vi "PreviewCell.vi"(6 "Current Variable settings":T2[](array[typedef]), 9 "Col header":string, 10 "Line Timing":T1, 11 "Cell contents":string) -> ()   [LabVIEW 2013]
uses:
  TypeDefs/Active procedure variables.ctl
  TypeDefs/LineTiming.ctl
  PackedLibraries/LuaEvaluatorAPI.lvlibp/API/t_Caching_Expression_Evaluator_Methods_Table.ctl
  PackedLibraries/LuaEvaluatorAPI.lvlibp
panel:
  out "parsed dt":dbl format="%#_6p"
  out "actual dt=t/steps":dbl format="%#_6p"
  in  "error in (no error)":errorcluster
  out "error out":errorcluster
  in  "Stand-Alone?":bool caption="This should NOT be set when VI called externally.\nIt is only included for debugging. (Caller list is checked and functions below won't be defined if not empty)."
  in  "User defined functions (IF Stand-Alone)":string="----------------------------------------\n-- The following functions are part of the \"standard load\" of functions and should not be messed with\n-- They are here for reference only.\n-- Please add any user functions above this comment\n-- -------------------------------------------------------------------------------------------\n\n-- Creates a linear ramp from A to B\nfunction LineRamp(f, Initial, Final)\n    return (1-f)*Initial + f*Final;\nend\n\n-- Creates an exponential ramp from A to B\nfunction ExpRamp(t, a, b, tau)\n   return (b - a*exp(tMax / tau) + (a-b)*exp(t/tau))/ ( 1 - exp(tMax / tau) );\nend\n\n-- Creates a sinewave\nfunction SinRamp(t,Offset,A,Freq, Phase)\n    return Offset + A * sin(2*pi*Freq*t + Phase)\nend\n\n-- Creates a blackman pulse\nfunction Blackman(f, Offset, A)\n    return Offset +  A*sqrt(0.5*cos(3.1415*(2*f-1))+0.08*cos(2*pi*(2*f-1))+0.42);\nend\n\n-- Creates a half-gauss ramp\nfunction HalfGaussRamp(t, a, b, Width)\n    local y;\n    y = exp(-(tMax^2)/Width^2);\n    y = (a -  b*y)/(1-y)  +  ((b-a)/(1-y))*exp(-((t-tMax)^2)/Width^2);\n    return y;\nend\n\n-- Creates an \"O'Hara\" ramp from A to B, for dipole evaporation\nfunction EvapRamp(t, a, b, tau)\n   local y;\n  y = log(a/b) / log(1+tMax/tau);\n  y = a * (1+t/tau)^(-y);\n  return y;\nend\n\n----------------------------------------------------------------\n\n\n-- Creates an exponential ramp from A to B in tEnd seconds\n-- useful for stopping a ramp at different times to measure T, N\nfunction ExpRampStep(t, a, b, tau, tEnd)\n   return (b - a*exp(tEnd / tau) + (a-b)*exp(t/tau))/ ( 1 - exp(tEnd / tau) );\nend\n\nfunction ExpRampEnd(tEv, a, b, tau, tEnd)\n   return (b - a*exp(tEnd / tau) + (a-b)*exp(tEv/tau))/ ( 1 - exp(tEnd / tau) );\nend\n\nfunction ExpRamp2(t,a,tau)\n   return a*exp(-t/tau)\nend\n\nfunction ExpRamp2End(tEnd,a,tau)\n   return a*exp(-tEnd/tau)\nend"
  out "y values":dbl[](array[numeric])
  out "x values":dbl[](array[numeric])
  out "Group enabled?":bool
  out "Cell contents":string
  out "Waveform Graph":waveform(dbl)(graph)
  # "useful to indicate (row,col)?"
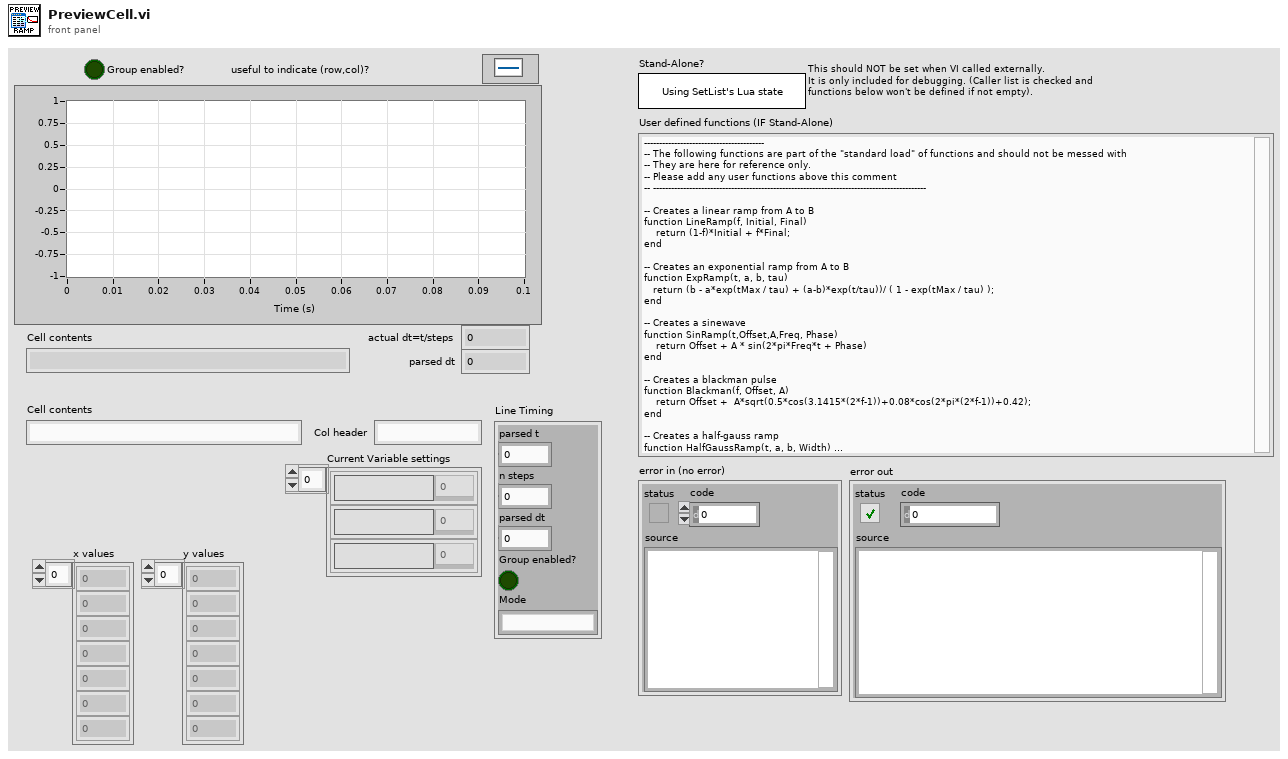
[diagram p1: front panel]
types:
  T1 = typedef "LineTiming.ctl" = cluster{"parsed t":dbl, "n steps":i32, "parsed dt":dbl, "Group enabled?":bool, "Mode":string}
  T2 = typedef "Active procedure variables.ctl" = cluster{"Procedure variable":string, "Value":dbl}
  T3 = typedef "LuaEvaluatorAPI.lvlibp/t_Caching_Expression_Evaluator_Methods_Table.ctl" = enum16{"set", "get", "eval", "assign", "isvalid", "execute", "evaltable", "close"}
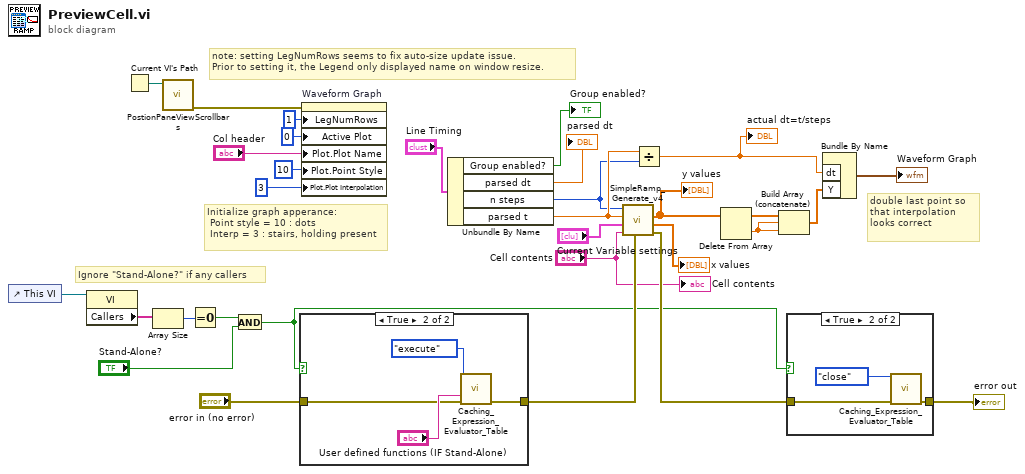
[diagram p0: block diagram]
diagram:
  # "note: setting LegNumRows seems to fix auto-size update issue.\nPrior to setting it, the Legend only displayed name on window resize."
  # "Ignore \"Stand-Alone?\" if any callers"
  # "Initialize graph apperance:\n Point style = 10 : dots\n Interp = 3 : stairs, holding present"
  # "double last point so that interpolation looks correct"
  n1 = control-ref of="This VI"() -> (w15:refnum<vi>)
  n2 = property class="VI"(reference=w15) -> ("Callers"=w14:string[])  [unwired: 1 in, 2 out]
  n3 = Current VI's Path() -> (path=w8:path)
  n4 = Array Size(array=w14) -> (size(s)=w13:i32)
  n5 = call "PostionPaneViewScrollbars.vi"("vi path"=w8) -> ("error out"=w7:errorcluster)  [unwired: 10 in]
  n6 = Equal To 0?(x=w13) -> (x = 0?=w12:bool)
  n7 = And(x=w12, y="Stand-Alone?") -> (x .and. y?=w10:bool)
  n8 = case shown="True" w10 {
    tunnel: [w32 w34] -> w29
    tunnel: "error in (no error)" -> [w32 w33]
    frame False {
    }
    frame True {
      n9 = call "Caching_Expression_Evaluator_Table.vi"("method"=t_Caching_Expression_Evaluator_Methods_Table."execute", "expression/scriptlet"="User defined functions (IF Stand-Alone)", "error in (no error)"=w33) -> ("error out"=w34:errorcluster)  [unwired: 10 in, 2 out]
    }
  }
  n10 = property on="Waveform Graph" class="WFGraph (strict)"(error in=w7, "LegNumRows"=u32 1 ("Active Plot"), "Active Plot"=u32 0, "Plot.Plot Name"="Col header", "Plot.Point Style"=u8 10, "Plot.Plot Interpolation"=u8 3) -> ()  [unwired: 1 in, 2 out]
  n11 = Unbundle By Name("Line Timing") -> ("Group enabled?"=→"Group enabled?":bool, "parsed dt"=→"parsed dt":dbl, "n steps"=w4:i32, "parsed t"=w5:dbl)
  n12 = call "SimpleRamp_Generate_v4.vi"("error in (no error)"=w29, "formula"="Cell contents", "Current Variable settings"="Current Variable settings", "ramp time"=w5, "Points"=w4) -> ("error out"=w28:errorcluster, "x values"=→"x values":dbl[], "y values"=w25:dbl[])  [unwired: 1 in, 1 out]
  "y values" <- w25
  n13 = Divide(x=w5, y=w4) -> (x/y=w26:dbl)
  "actual dt=t/steps" <- w26
  n14 = Delete From Array(array=w25) -> (deleted portion=w23:dbl, array with subset deleted=w24:dbl[])  [unwired: 2 in]
  n15 = Build Array (concatenate)(w24, w23, w23) -> (w22:dbl[])
  n16 = case shown="True" w10 {
    tunnel: w28 -> [w37 w39]
    tunnel: [w37 w38] -> w16
    frame False {
    }
    frame True {
      n17 = call "Caching_Expression_Evaluator_Table.vi"("method"=t_Caching_Expression_Evaluator_Methods_Table."close", "error in (no error)"=w39) -> ("error out"=w38:errorcluster)  [unwired: 11 in, 2 out]
    }
  }
  "error out" <- w16
  n18 = Bundle By Name("dt"=w26, "Y"=w22) -> (→"Waveform Graph":waveform(dbl))  [unwired: 1 in]
  "Cell contents" <- "Cell contents"
